vi "Index_Array.vi"(0 "E or S Index Array":T1, 1 "Choose Index Array":T2, 5 "Index 1D":i32, 7 "Index Array 1D":i8[](array[numeric])=[1, 3, 4, -2, 0, 10], 9 "Indexs Array 2D":T3={"Rows"=-1, "Columns"=-1} {"Columns" min=-1; "Rows" min=-1}, 11 "Index Array 2D":i8[][](array[numeric])=[[0, 4, -3], [1, 5, -4], [2, -1, -5], [3, -2, 100]]) -> (6 "Index Value":i8, 10 "Index SubArray":i8[](array[numeric]))   [LabVIEW 2018]
uses:
  Controls/Rows_Columns.ctl
  Controls/1D_2D.ctl
  Controls/E_S.ctl
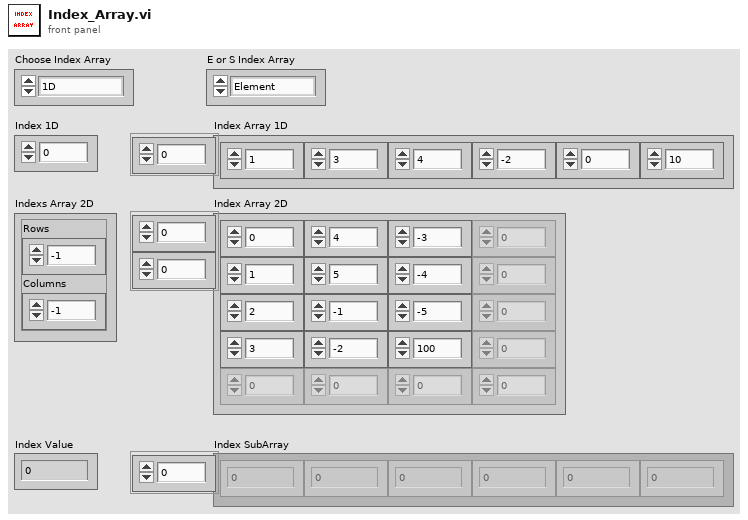
[diagram p1: front panel]
types:
  T1 = typedef "E_S.ctl" = enum16{"Element", "SubArray"}
  T2 = typedef "1D_2D.ctl" = enum16{"1D", "2D"}
  T3 = typedef "Rows_Columns.ctl" = cluster{"Rows":i32, "Columns":i32}
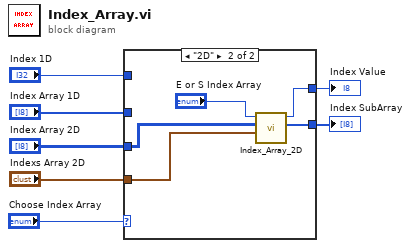
[diagram p0: block diagram]
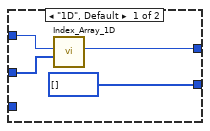
[diagram p2: hidden frame]
diagram:
  n1 = case shown="\"2D\"" "Choose Index Array" {
    tunnel: "Index 1D" -> [w11 _]
    tunnel: "Index Array 1D" -> [w10 _]
    tunnel: [w9 w16] -> w5
    tunnel: "Indexs Array 2D" -> [_ w14]
    tunnel: "Index Array 2D" -> [_ w13]
    tunnel: [i8[] [] ("SubArray") w15] -> w2
    frame "1D", Default {
      n2 = call "Index_Array_1D.vi"("Index Array 1D"=w10, "Index"=w11) -> ("Value"=w9:i8)  [unwired: 9 in]
    }
    frame "2D" {
      n3 = call "Index_Array_2D.vi"("Indexs IA"=w14, "Index Array 2D"=w13, "E or S Index Array 2D"="E or S Index Array") -> ("Index SubArray"=w15:i8[], "Index Value"=w16:i8)  [unwired: 7 in]
    }
  }
  "Index Value" <- w5
  "Index SubArray" <- w2
